vi "GV pretrigger.vi"() -> ()   [LabVIEW 2017]
panel:
  out "Pretrigger":bool
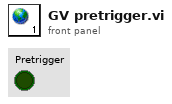
[diagram p1: front panel]
diagram:
